vi "4Pi Drift Monitor.vi"() -> ()   [LabVIEW 2016]
uses:
  <vilib>/vision/Image Controls.llb/IMAQ Image.ctl
  4Pi Drift Monitor Controls/4Pi Drift Monitor - Notifier Type.ctl
  4Pi Drift Monitor Controls/4Pi Drift Monitor - Actions.ctl
  Hardware Configuration/Hardware Configuration Controls/Device Type.ctl
  Hardware Configuration/Hardware Configuration Controls/Device Function.ctl
panel:
  in  "CCD Offset":dbl=100.0
  in  "Offset Position Scale":dbl=2.0
  out "ROI Stack":u16[][][](array[numeric])
  out "Y (nm)":cluster{dbl, dbl, dbl, dbl}(graph)
  in  "Quit":bool
  out "Init X pos (px)":dbl[](array[numeric])
  out "Init Y pos (px)":dbl[](array[numeric])
  out "Y pos (px)":dbl[](array[numeric])
  out "X pos (px)":dbl[](array[numeric])
  in  "Frame Accumulation":i32
  in  "ROI Size":i32=7
  in  "Camera Px. Size (nm)":dbl=0.1
  in  "qd4":bool=TRUE
  in  "qd3":bool=TRUE
  in  "qd2":bool=TRUE
  in  "qd1":bool=TRUE
  out "X (nm)":cluster{dbl, dbl, dbl, dbl}(graph)
  in  "Start Monitor":bool
  # "Quadrant"
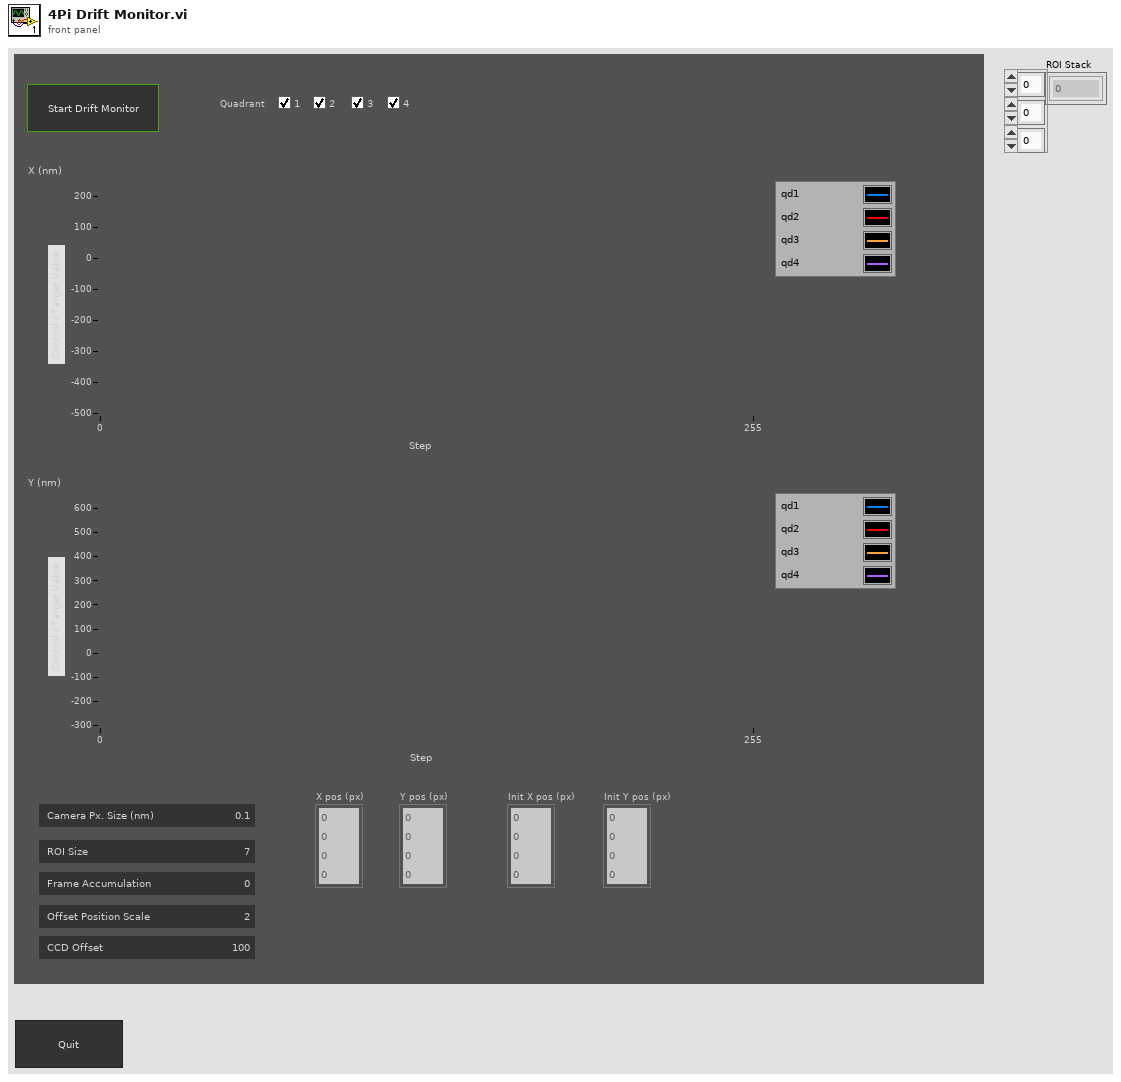
[diagram p1: front panel]
types:
  T1 = typedef "4Pi Drift Monitor - Actions.ctl" = enum16{"Idle", "Start Monitor", "Get Initial XY Pos", "Get Initial Image", "Get Image", "Get XY Position", "Update Plots", "Exit Loop", "Abort", "Quit"}
  T2 = typedef "4Pi Drift Monitor - Notifier Type.ctl" = cluster{"Action":T1, "Frame Accums.":u16, "Camera Px. Size (nm)":dbl, "QD On/Off":bool[], "Image Ref":T3[], "ROI Size":i32, "Frame Accumulation":u16, "ROI Stack":u16[][][], "Running?":bool}
  T3 = typedef "IMAQ Image.ctl" = refnum<image>
  T4 = typedef "Device Function.ctl" = enum16{"Primary", "Secondary", "Overview", "Wide Field Drift Correction", "642 nm Excitation", "560 nm Excitation", "546 nm Excitation", "488 nm Excitation", "405 nm Excitation", "Objective Drift Correction", "4Pi Objective Lock", "Objective XY", "Objective Z", "Sample XY", "Sample Coarse Z", "Sample Z", "4Pi Lower", "4Pi Upper", "Adj Cavity", "Line Scanning", "Alert"}
  T5 = typedef "Device Type.ctl" = enum16{"AOTF", "Camera", "Deformable Mirror", "Laser", "Shutter", "Stage", "Waveform", "Email"}
  T6 = typedef "4Pi DCM-2D Gaussian - Best Fit Parameters.ctl" = cluster{"Amplitude":dbl, "X Position":dbl, "Y Position":dbl, "X Width":dbl, "Y Width":dbl, "Offset":dbl}
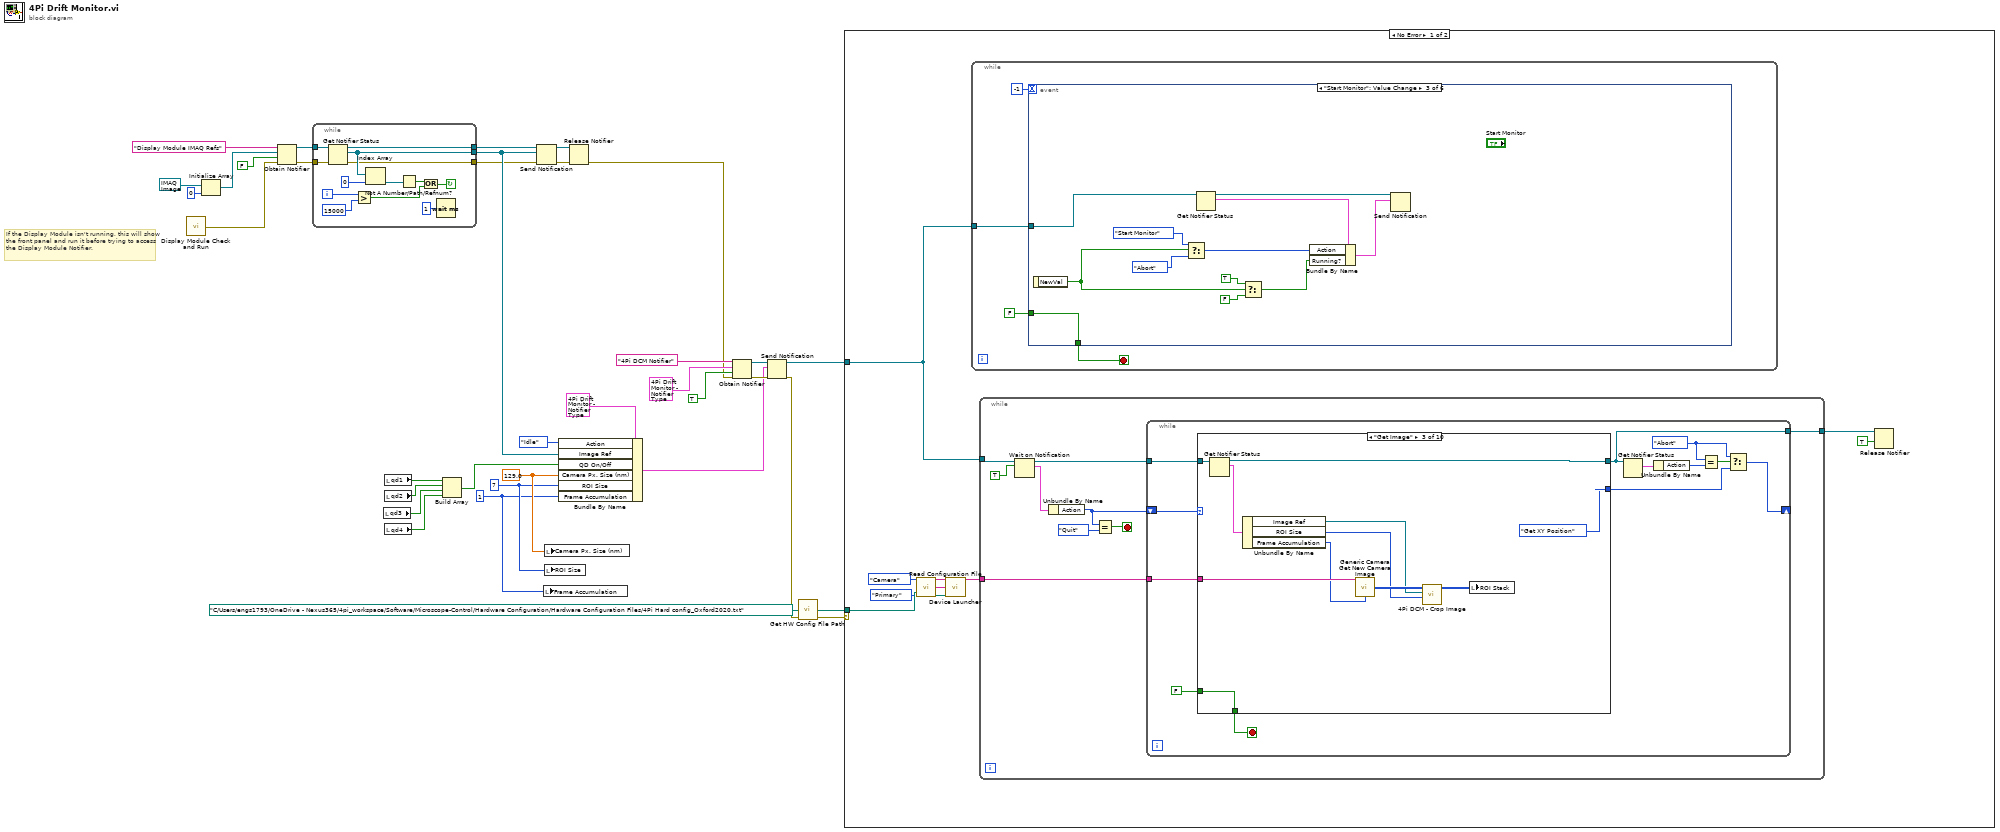
[diagram p0: block diagram]
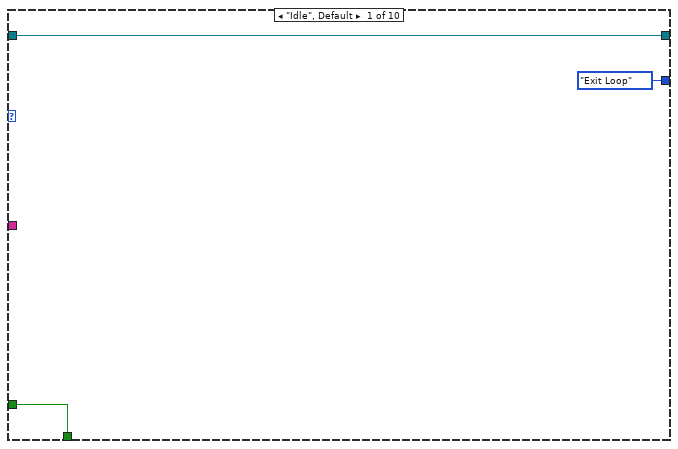
[diagram p2: hidden frame]
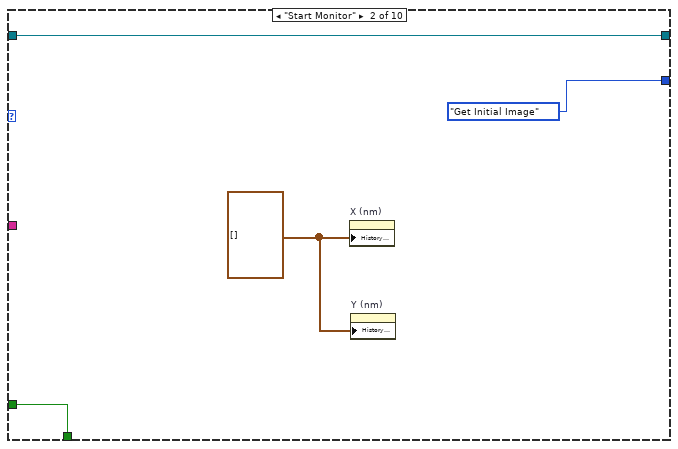
[diagram p3: hidden frame]
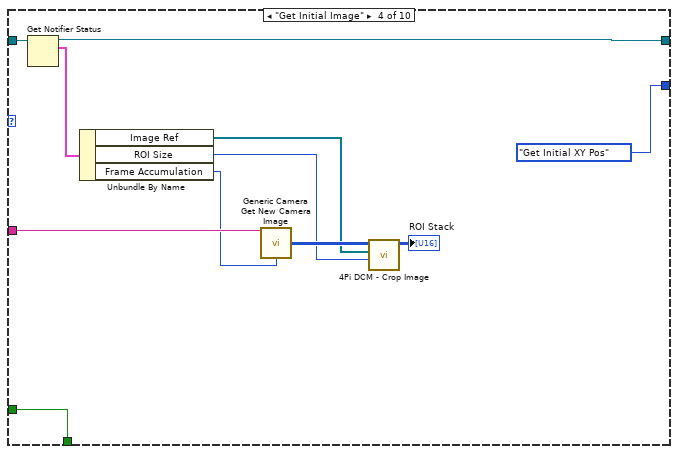
[diagram p4: hidden frame]
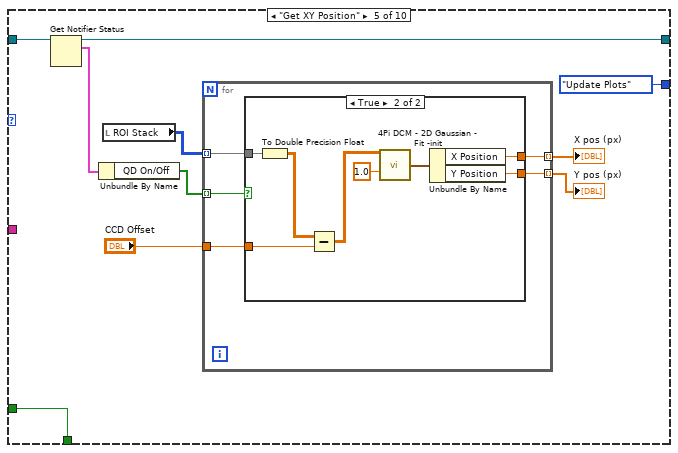
[diagram p5: hidden frame]
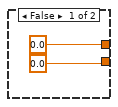
[diagram p6: hidden frame]
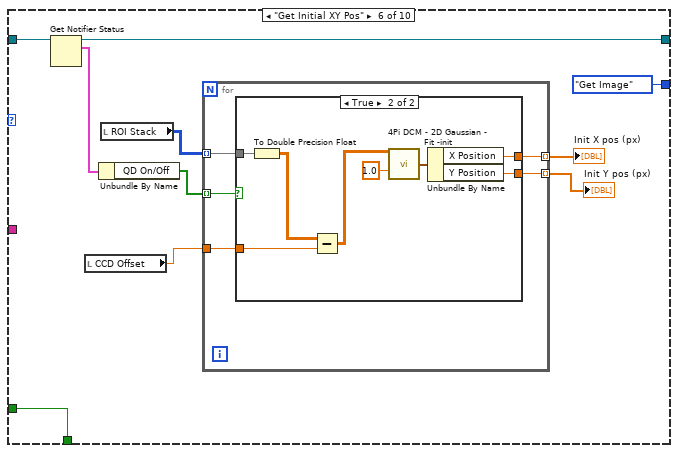
[diagram p7: hidden frame]
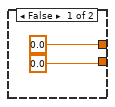
[diagram p8: hidden frame]
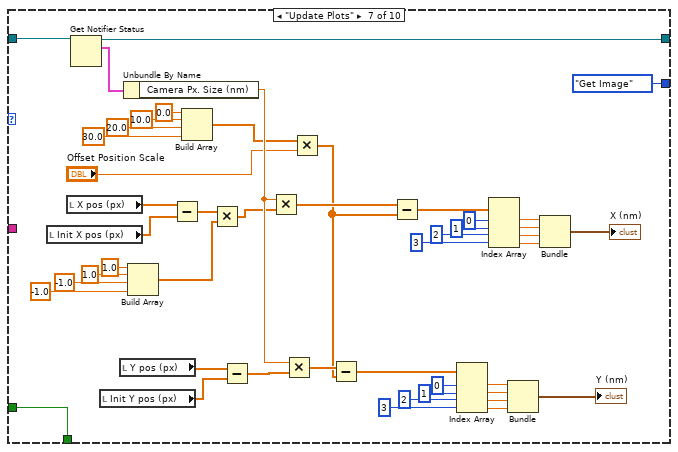
[diagram p9: hidden frame]
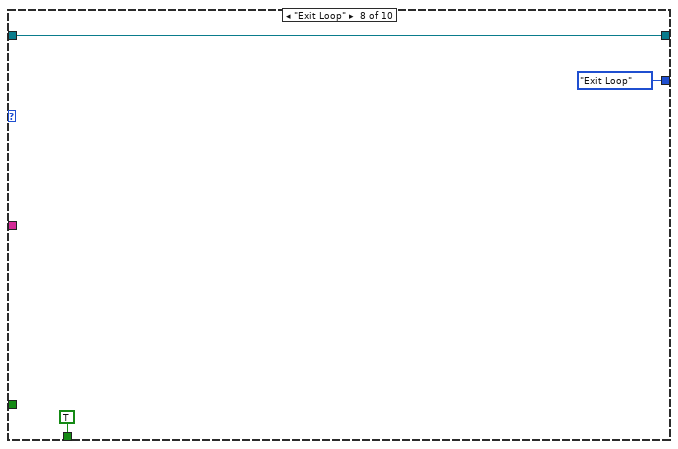
[diagram p10: hidden frame]
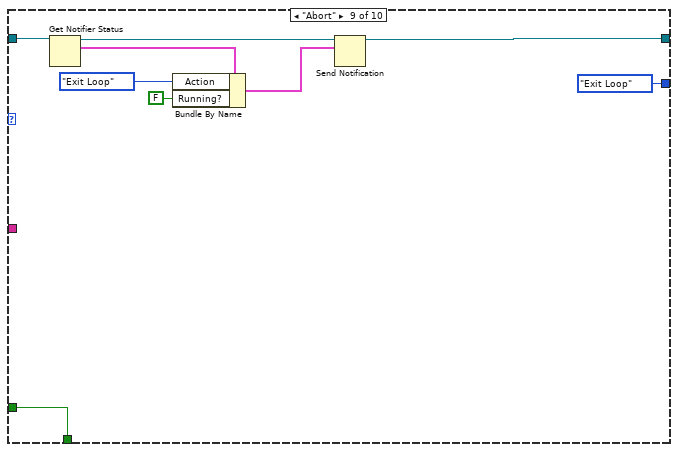
[diagram p11: hidden frame]
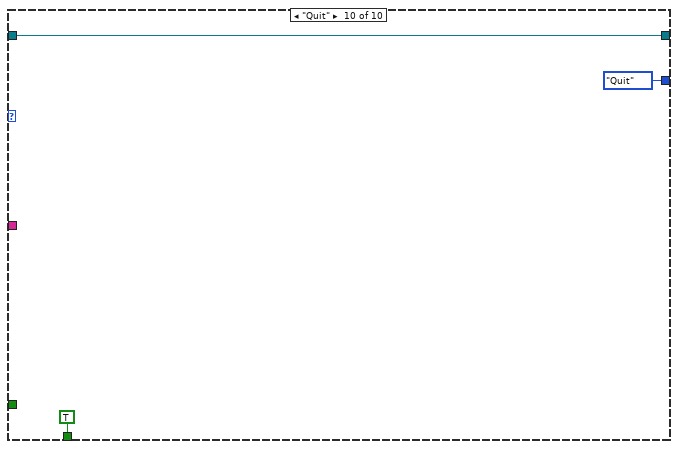
[diagram p12: hidden frame]
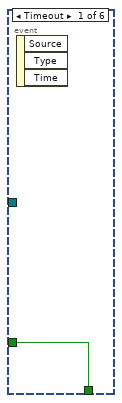
[diagram p13: hidden frame]
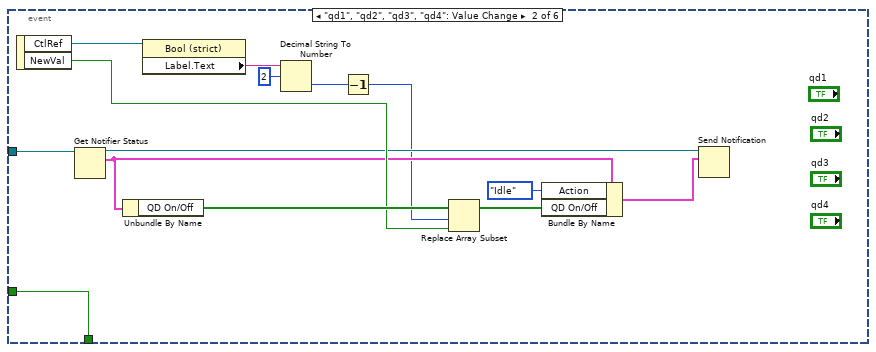
[diagram p14: hidden frame]
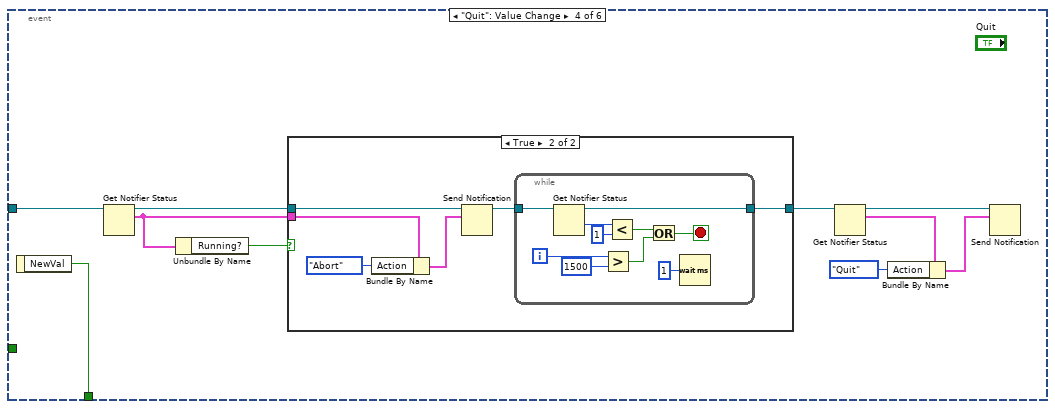
[diagram p15: hidden frame]
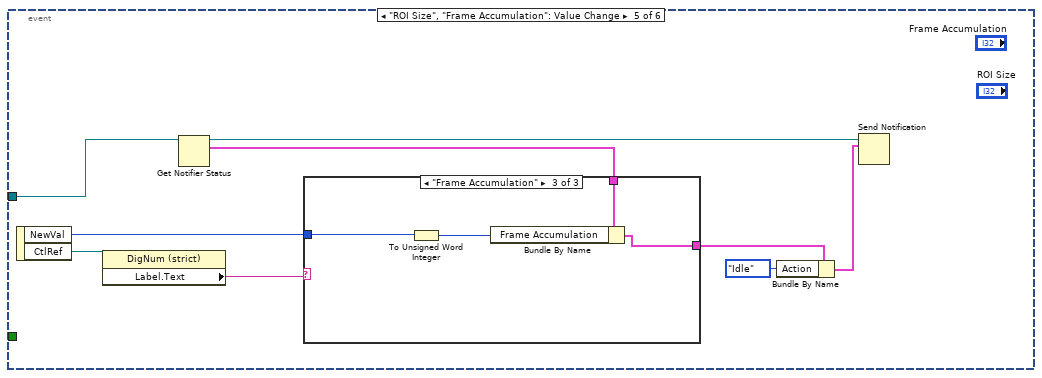
[diagram p17: hidden frame]
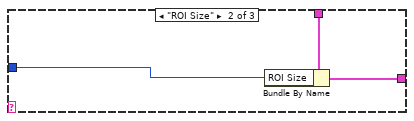
[diagram p19: hidden frame]
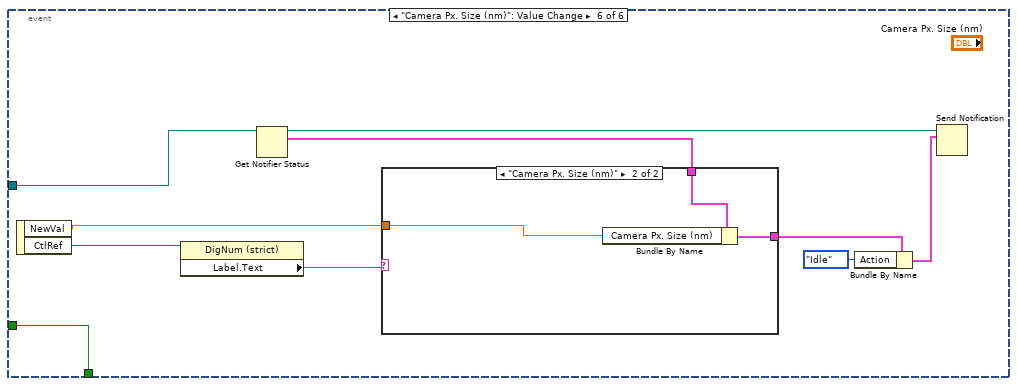
[diagram p20: hidden frame]
diagram:
  w2 = u16 1 ("Frame Accumulation")
  w3 = 7 ("ROI Size")
  w4 = 129.0 ("Camera Px. Size (nm)")
  # "If the Display Module isn't running, this will show the front panel and run it before trying to access the Display Module Notifier."
  n1 = call "Display Module Check and Run.vi"() -> ("Error"=w31:errorcluster)  [unwired: 15 in]
  n2 = Initialize Array(T3 refnum ("New Image"), 0 ("dimension size")) -> (w28:T3[])
  n3 = Obtain Notifier(name (unnamed)="Display Module IMAQ Refs", notification data type=w28, create if not found? (T)=FALSE, error in (no error)=w31) -> (notifier out=w30:refnum<notifier>, error out=w29:errorcluster)  [unwired: 1 out]
  n4 = while {
    tunnel: w30 -> [w48]
    tunnel: w29 -> [w47]
    tunnel: [w46] -> w8
    tunnel: [w45] -> w7
    tunnel: [w41] -> w6
    i -> [w40]
    stop <- w37 continue-if-true
    n5 = Get Notifier Status(notifier=w48, error in (no error)=w47) -> (notifier out=w46:refnum<notifier>, current notification=w45:T3[], error out=w41:errorcluster)  [unwired: 2 out]
    n6 = Greater?(x=w40, y=15000) -> (0:w36:bool)
    n7 = Index Array(array=w45, index=0) -> (element=w43:T3)
    n8 = Not A Number/Path/Refnum?(number/path/refnum=w43) -> (NaN/Path/Refnum?=w38:bool)
    n9 = Or(x=w38, y=w36) -> (x .or. y?=w37:bool)
    n10 = Wait (ms)(milliseconds to wait=u32 1) -> ()  [unwired: 1 out]
  }
  n11 = local read "qd3"() -> (w13:bool)
  n12 = local read "qd1"() -> (w15:bool)
  n13 = local read "qd2"() -> (w14:bool)
  n14 = local read "qd4"() -> (w12:bool)
  n15 = Build Array(w15, w14, w13, w12) -> (w11:bool[])
  n16 = Send Notification(notification=w7, notifier=w8, error in (no error)=w6) -> (notifier out=w9:refnum<notifier>, error out=w10:errorcluster)
  n17 = local write "Frame Accumulation"(w2) -> ()
  n18 = local write "Camera Px. Size (nm)"(w4) -> ()
  n19 = local write "ROI Size"(w3) -> ()
  n20 = Bundle By Name(cluster=T2 {"Action"=enum."Start Monitor", "Frame Accums."=0, "Camera Px. Size (nm)"=0.1, "QD On/Off"=[], "Image Ref"=[], "ROI Size"=0, "Frame Accumulation"=0, "ROI Stack"=[], "Running?"=FALSE} ("4Pi Drift Monitor Notifier Type"), "Action"=4Pi_Drift_Monitor_-_Actions."Idle", "Image Ref"=w7, "QD On/Off"=w11, "Camera Px. Size (nm)"=w4, "ROI Size"=w3, "Frame Accumulation"=w2) -> (w17:T2)
  n21 = Release Notifier(notifier=w9, error in (no error)=w10) -> (error out=w5:errorcluster)  [unwired: 1 in, 2 out]
  n22 = Obtain Notifier(name (unnamed)="4Pi DCM Notifier", notification data type=T2 {"Action"=enum."Start Monitor", "Frame Accums."=0, "Camera Px. Size (nm)"=0.1, "QD On/Off"=[], "Image Ref"=[], "ROI Size"=0, "Frame Accumulation"=0, "ROI Stack"=[], "Running?"=FALSE} ("4Pi Drift Monitor Notifier Type"), create if not found? (T)=TRUE, error in (no error)=w5) -> (notifier out=w25:refnum<notifier>, error out=w23:errorcluster)  [unwired: 1 out]
  n23 = Send Notification(notification=w17, notifier=w25, error in (no error)=w23) -> (notifier out=w16:refnum<notifier>, error out=w22:errorcluster)
  n24 = call "Get HW Config File Path.vi"("File Path"=path "C:/Users/engs1793/OneDrive - Nexus365/4pi_workspace/Software/Microscope-Control/Hardware Configuration/Hardware Configuration Files/4Pi Hard config_Oxford2020.txt", "Error"=w22) -> ("File Path"=w20:path, "Error"=w21:errorcluster)  [unwired: 12 in]
  n25 = case shown="No Error" w21 {
    tunnel: w20 -> [w55 _]
    tunnel: w16 -> [w51 _]
    frame No Error {
      n26 = call "Read Configuration File.vi"("Device Type"=Device_Type."Camera", "Device Function"=Device_Function."Primary", "Config File Path"=w55) -> ("Unique Notifier Name"=w56:string, "Device Ports/IDs/Channels"=w58:string[], "Device Engine Path"=w57:path)  [unwired: 9 in, 1 out]
      n27 = call "Device Launcher.vi"("Notifier Name"=w56, "Device Ports/IDs/Channels"=w58, "Device Engine Path"=w57) -> ("Notifier Name"=w52:string)  [unwired: 11 in, 1 out]
      n28 = while {
        tunnel: w51 -> [w224]
        stop <- w223 stop-if-true
        n29 = event shown="[2] \"Start Monitor\": Value Change" {
          selector: _ -> [_ _ _ _ _ _]
          dyn-events: _ -> [_ _ _ _ _ _]
          timeout: -1 -> [_ _ _ _ _ _]
          tunnel: w224 -> [_ w238 w242 w253 w285 w296]
          tunnel: [w225 w228 w245 w261 _ w305] -> w223
          tunnel: FALSE -> [w225 w228 w245 _ _ w305]
          event Timeout {
            n30 = event-data() -> ()  [unwired: 1 in, 3 out]
          }
          event "qd1", "qd2", "qd3", "qd4": Value Change {
            n31 = event-data() -> ("CtlRef"=w239:refnum<vi>, "NewVal"=w234:bool)  [unwired: 1 in]
            n32 = Get Notifier Status(notifier=w238) -> (notifier out=w230:refnum<notifier>, current notification=w233:T2)  [unwired: 1 in, 3 out]
            n33 = Unbundle By Name(w233) -> ("QD On/Off"=w237:bool[])
            n34 = property class="Bool (strict)"(reference=w239) -> ("Label.Text"=w236:string)  [unwired: 1 in, 2 out]
            n35 = Decimal String To Number(string=w236, offset=2 ("offset (0)")) -> (number=w227:i32)  [unwired: 1 in, 1 out]
            n36 = Decrement(x=w227) -> (x-1=w226:i32)
            n37 = Replace Array Subset(array=w237, new element=w234, index=w226) -> (w232:bool[])
            n38 = Bundle By Name(cluster=w233, "Action"=4Pi_Drift_Monitor_-_Actions."Idle", "QD On/Off"=w232) -> (w231:T2)
            n39 = Send Notification(notification=w231, notifier=w230) -> ()  [unwired: 1 in, 2 out]
          }
          event "Start Monitor": Value Change {
            n40 = event-data() -> ("NewVal"=w241:bool)  [unwired: 1 in]
            n41 = Select(t=4Pi_Drift_Monitor_-_Actions."Start Monitor" ("Action"), s=w241, f=4Pi_Drift_Monitor_-_Actions."Abort") -> (s? t:f=w248:T1)
            n42 = Get Notifier Status(notifier=w242) -> (notifier out=w246:refnum<notifier>, current notification=w251:T2)  [unwired: 1 in, 3 out]
            n43 = Select(t=TRUE ("Running?"), s=w241, f=FALSE) -> (s? t:f=w240:bool)
            n44 = Bundle By Name(cluster=w251, "Action"=w248, "Running?"=w240) -> (w247:T2)
            n45 = Send Notification(notification=w247, notifier=w246) -> ()  [unwired: 1 in, 2 out]
          }
          event "Quit": Value Change {
            n46 = event-data() -> ("NewVal"=w261:bool)  [unwired: 1 in]
            n47 = Get Notifier Status(notifier=w253) -> (notifier out=w256:refnum<notifier>, current notification=w254:T2)  [unwired: 1 in, 3 out]
            n48 = Unbundle By Name(w254) -> ("Running?"=w257:bool)
            n49 = case shown="True" w257 {
              tunnel: w256 -> [w262 w267]
              tunnel: [w262 w264] -> w255
              tunnel: w254 -> [_ w268]
              frame False {
              }
              frame True {
                n50 = Bundle By Name(cluster=w268, "Action"=4Pi_Drift_Monitor_-_Actions."Abort") -> (w266:T2)
                n51 = Send Notification(notification=w266, notifier=w267) -> (notifier out=w265:refnum<notifier>)  [unwired: 1 in, 1 out]
                n52 = while {
                  tunnel: w265 -> [w278]
                  tunnel: [w273] -> w264
                  i -> [w272]
                  stop <- w274 stop-if-true
                  n53 = Get Notifier Status(notifier=w278) -> (notifier out=w273:refnum<notifier>, # waiting=w277:i32)  [unwired: 1 in, 3 out]
                  n54 = Greater?(x=w272, y=1500) -> (0:w270:bool)
                  n55 = Less?(x=w277, y=1) -> (x < y?=w275:bool)
                  n56 = Or(x=w275, y=w270) -> (x .or. y?=w274:bool)
                  n57 = Wait (ms)(milliseconds to wait=u32 1) -> ()  [unwired: 1 out]
                }
              }
            }
            n58 = Get Notifier Status(notifier=w255) -> (notifier out=w259:refnum<notifier>, current notification=w260:T2)  [unwired: 1 in, 3 out]
            n59 = Bundle By Name(cluster=w260, "Action"=4Pi_Drift_Monitor_-_Actions."Quit") -> (w258:T2)
            n60 = Send Notification(notification=w258, notifier=w259) -> ()  [unwired: 1 in, 2 out]
          }
          event "ROI Size", "Frame Accumulation": Value Change {
            n61 = event-data() -> ("NewVal"=w283:i32, "CtlRef"=w287:refnum<vi>)  [unwired: 1 in]
            n62 = property class="DigNum (strict)"(reference=w287) -> ("Label.Text"=w286:string)  [unwired: 1 in, 2 out]
            n63 = Get Notifier Status(notifier=w285) -> (notifier out=w282:refnum<notifier>, current notification=w284:T2)  [unwired: 1 in, 3 out]
            n64 = case shown="\"Frame Accumulation\"" w286 {
              tunnel: w284 -> [w288 w291 w295]
              tunnel: w283 -> [_ w290 w293]
              tunnel: [w288 w289 w294] -> w281
              frame Default {
              }
              frame "ROI Size" {
                n65 = Bundle By Name(cluster=w291, "ROI Size"=w290) -> (w289:T2)
              }
              frame "Frame Accumulation" {
                n66 = To Unsigned Word Integer(number=w293) -> (unsigned 16bit integer=w292:u16)
                n67 = Bundle By Name(cluster=w295, "Frame Accumulation"=w292) -> (w294:T2)
              }
            }
            n68 = Bundle By Name(cluster=w281, "Action"=4Pi_Drift_Monitor_-_Actions."Idle") -> (w279:T2)
            n69 = Send Notification(notification=w279, notifier=w282) -> ()  [unwired: 1 in, 2 out]
          }
          event "Camera Px. Size (nm)": Value Change {
            n70 = event-data() -> ("NewVal"=w297:dbl, "CtlRef"=w298:refnum<vi>)  [unwired: 1 in]
            n71 = property class="DigNum (strict)"(reference=w298) -> ("Label.Text"=w304:string)  [unwired: 1 in, 2 out]
            n72 = Get Notifier Status(notifier=w296) -> (notifier out=w302:refnum<notifier>, current notification=w303:T2)  [unwired: 1 in, 3 out]
            n73 = case shown="\"Camera Px. Size (nm)\"" w304 {
              tunnel: w303 -> [w306 w309]
              tunnel: w297 -> [_ w308]
              tunnel: [w306 w307] -> w301
              frame Default {
              }
              frame "Camera Px. Size (nm)" {
                n74 = Bundle By Name(cluster=w309, "Camera Px. Size (nm)"=w308) -> (w307:T2)
              }
            }
            n75 = Bundle By Name(cluster=w301, "Action"=4Pi_Drift_Monitor_-_Actions."Idle") -> (w299:T2)
            n76 = Send Notification(notification=w299, notifier=w302) -> ()  [unwired: 1 in, 2 out]
          }
        }
      }
      n77 = while {
        tunnel: w52 -> [w61]
        tunnel: w51 -> [w65]
        tunnel: [w59] -> w49
        stop <- w63 stop-if-true
        n78 = Wait on Notification(notifier=w65, ignore previous (F)=TRUE) -> (notifier out=w62:refnum<notifier>, notification=w66:T2)  [unwired: 2 in, 2 out]
        n79 = Unbundle By Name(w66) -> ("Action"=w60:T1)
        n80 = Equal?(x=w60, y=4Pi_Drift_Monitor_-_Actions."Quit") -> (x = y?=w63:bool)
        n81 = while {
          tunnel: w62 -> [w79]
          tunnel: w61 -> [w78]
          shift-right: [w72] -> _
          shift-left: w60 -> [w71]
          tunnel: [w68] -> w59
          stop <- w70 stop-if-true
          w74 = 4Pi_Drift_Monitor_-_Actions."Abort" ("x")
          n82 = case shown="\"Get Image\"" w71 {
            tunnel: [w81 w86 w88 w99 w113 w138 w179 w208 w211 w218] -> w68
            tunnel: w79 -> [w81 w86 w97 w108 w118 w143 w205 w208 w217 w218]
            tunnel: w78 -> [_ _ w96 w107 _ _ _ _ _ _]
            tunnel: [4Pi_Drift_Monitor_-_Actions."Exit Loop" ("y") 4Pi_Drift_Monitor_-_Actions."Get Initial Image" ("y") 4Pi_Drift_Monitor_-_Actions."Get XY Position" ("y") 4Pi_Drift_Monitor_-_Actions."Get Initial XY Pos" ("y") 4Pi_Drift_Monitor_-_Actions."Update Plots" ("y") 4Pi_Drift_Monitor_-_Actions."Get Image" ("y") 4Pi_Drift_Monitor_-_Actions."Get Image" ("y") 4Pi_Drift_Monitor_-_Actions."Exit Loop" ("y") 4Pi_Drift_Monitor_-_Actions."Exit Loop" ("y") 4Pi_Drift_Monitor_-_Actions."Quit" ("y")] -> w73
            tunnel: [w80 w83 w89 w100 w112 w137 w178 TRUE w210 TRUE] -> w70
            tunnel: FALSE -> [w80 w83 w89 w100 w112 w137 w178 _ w210 _]
            frame "Idle", Default {
            }
            frame "Start Monitor" {
              w84 = cluster{dbl, dbl, dbl, dbl}[] [] ("History Data")
              n83 = property on="X (nm)" class="WFChart (strict)"("History Data"=w84) -> ()  [unwired: 2 in, 2 out]
              n84 = property on="Y (nm)" class="WFChart (strict)"("History Data"=w84) -> ()  [unwired: 2 in, 2 out]
            }
            frame "Get Image" {
              n85 = Get Notifier Status(notifier=w97) -> (notifier out=w88:refnum<notifier>, current notification=w91:T2)  [unwired: 1 in, 3 out]
              n86 = Unbundle By Name(w91) -> ("Image Ref"=w94:T3[], "ROI Size"=w93:i32, "Frame Accumulation"=w92:u16)
              n87 = call "Generic Camera Get New Camera Image.vi"("Camera Notifier Name"=w96, "Frames"=w92) -> ("Image - U16"=w95:u16[][])  [unwired: 11 in, 2 out]
              n88 = call "4Pi DCM - Crop Image.vi"("ROI Size"=w93, "Image Refs"=w94, "Input Image (U16)"=w95) -> ("Output Image Stack"=w87:u16[][][])  [unwired: 8 in]
              n89 = local write "ROI Stack"(w87) -> ()
            }
            frame "Get Initial Image" {
              n90 = Get Notifier Status(notifier=w108) -> (notifier out=w99:refnum<notifier>, current notification=w102:T2)  [unwired: 1 in, 3 out]
              n91 = Unbundle By Name(w102) -> ("Image Ref"=w105:T3[], "ROI Size"=w104:i32, "Frame Accumulation"=w103:u16)
              n92 = call "Generic Camera Get New Camera Image.vi"("Camera Notifier Name"=w107, "Frames"=w103) -> ("Image - U16"=w106:u16[][])  [unwired: 11 in, 2 out]
              n93 = call "4Pi DCM - Crop Image.vi"("ROI Size"=w104, "Image Refs"=w105, "Input Image (U16)"=w106) -> ("Output Image Stack"=→"ROI Stack":u16[][][])  [unwired: 8 in]
            }
            frame "Get XY Position" {
              n94 = Get Notifier Status(notifier=w118) -> (notifier out=w113:refnum<notifier>, current notification=w117:T2)  [unwired: 1 in, 3 out]
              n95 = Unbundle By Name(w117) -> ("QD On/Off"=w111:bool[])
              n96 = local read "ROI Stack"() -> (w110:u16[][][])
              n97 = for {
                tunnel: w110 -> [w123] mode=indexing
                tunnel: [w122] -> w116 mode=indexing
                tunnel: [w121] -> w115 mode=indexing
                tunnel: w111 -> [w120] mode=indexing
                tunnel: "CCD Offset" -> [w119]
                n98 = case shown="True" w120 {
                  tunnel: w123 -> [_ w133]
                  tunnel: [0.0 ("X Position") w130] -> w122
                  tunnel: [0.0 ("Y Position") w129] -> w121
                  tunnel: w119 -> [_ w127]
                  frame False {
                  }
                  frame True {
                    n99 = To Double Precision Float(number=w133) -> (double precision float=w128:dbl[][])
                    n100 = Subtract(x=w128, y=w127) -> (x-y=w126:dbl[][])
                    n101 = call "4Pi DCM - 2D Gaussian - Fit -init.vi"("Image In (DBL)"=w126, "width"=1.0) -> ("Best Fit Params"=w131:T6)  [unwired: 12 in, 1 out]
                    n102 = Unbundle By Name(w131) -> ("X Position"=w130:dbl, "Y Position"=w129:dbl)
                  }
                }
              }
              "X pos (px)" <- w116
              "Y pos (px)" <- w115
            }
            frame "Get Initial XY Pos" {
              n103 = Get Notifier Status(notifier=w143) -> (notifier out=w138:refnum<notifier>, current notification=w142:T2)  [unwired: 1 in, 3 out]
              n104 = local read "CCD Offset"() -> (w134:dbl)
              n105 = Unbundle By Name(w142) -> ("QD On/Off"=w136:bool[])
              n106 = local read "ROI Stack"() -> (w135:u16[][][])
              n107 = for {
                tunnel: w135 -> [w148] mode=indexing
                tunnel: [w147] -> w141 mode=indexing
                tunnel: [w146] -> w140 mode=indexing
                tunnel: w136 -> [w145] mode=indexing
                tunnel: w134 -> [w144]
                n108 = case shown="True" w145 {
                  tunnel: w148 -> [_ w158]
                  tunnel: [0.0 ("X Position") w155] -> w147
                  tunnel: [0.0 ("Y Position") w154] -> w146
                  tunnel: w144 -> [_ w152]
                  frame False {
                  }
                  frame True {
                    n109 = To Double Precision Float(number=w158) -> (double precision float=w153:dbl[][])
                    n110 = Subtract(x=w153, y=w152) -> (x-y=w151:dbl[][])
                    n111 = call "4Pi DCM - 2D Gaussian - Fit -init.vi"("Image In (DBL)"=w151, "width"=1.0) -> ("Best Fit Params"=w156:T6)  [unwired: 12 in, 1 out]
                    n112 = Unbundle By Name(w156) -> ("X Position"=w155:dbl, "Y Position"=w154:dbl)
                  }
                }
              }
              "Init X pos (px)" <- w141
              "Init Y pos (px)" <- w140
            }
            frame "Update Plots" {
              n113 = local read "Init X pos (px)"() -> (w202:dbl[])
              n114 = local read "X pos (px)"() -> (w203:dbl[])
              n115 = Get Notifier Status(notifier=w205) -> (notifier out=w179:refnum<notifier>, current notification=w204:T2)  [unwired: 1 in, 3 out]
              n116 = local read "Init Y pos (px)"() -> (w199:dbl[])
              n117 = local read "Y pos (px)"() -> (w200:dbl[])
              n118 = Unbundle By Name(w204) -> ("Camera Px. Size (nm)"=w198:dbl)
              n119 = Build Array(1.0 ("element"), 1.0 ("element"), -1.0 ("element"), -1.0 ("element")) -> (w160:dbl[])
              n120 = Subtract(x=w203, y=w202) -> (x-y=w161:dbl[])
              n121 = Build Array(0.0 ("element"), 10.0 ("element"), 20.0 ("element"), 30.0 ("element")) -> (w172:dbl[])
              n122 = Multiply(x=w161, y=w160) -> (x*y=w159:dbl[])
              n123 = Subtract(x=w200, y=w199) -> (x-y=w201:dbl[])
              n124 = Multiply(x=w198, y=w159) -> (x*y=w168:dbl[])
              n125 = Multiply(x=w198, y=w201) -> (x*y=w169:dbl[])
              n126 = Multiply(x=w172, y="Offset Position Scale") -> (x*y=w166:dbl[])
              n127 = Subtract(x=w169, y=w166) -> (x-y=w167:dbl[])
              n128 = Subtract(x=w168, y=w166) -> (x-y=w170:dbl[])
              n129 = Index Array(array=w167, index #1=0 ("index"), index #2=1 ("index"), index #3=2 ("index"), index #4=3 ("index")) -> (element #1=w185:dbl, element #2=w184:dbl, element #3=w183:dbl, element #4=w182:dbl)
              n130 = Index Array(array=w170, index #1=0 ("index"), index #2=1 ("index"), index #3=2 ("index"), index #4=3 ("index")) -> (element #1=w193:dbl, element #2=w192:dbl, element #3=w191:dbl, element #4=w190:dbl)
              n131 = Bundle(w185, w184, w183, w182) -> (→"Y (nm)":cluster{dbl, dbl, dbl, dbl})  [unwired: 1 in]
              n132 = Bundle(w193, w192, w191, w190) -> (→"X (nm)":cluster{dbl, dbl, dbl, dbl})  [unwired: 1 in]
            }
            frame "Exit Loop" {
            }
            frame "Abort" {
              n133 = Get Notifier Status(notifier=w217) -> (notifier out=w216:refnum<notifier>, current notification=w215:T2)  [unwired: 1 in, 3 out]
              n134 = Bundle By Name(cluster=w215, "Action"=4Pi_Drift_Monitor_-_Actions."Exit Loop", "Running?"=FALSE) -> (w214:T2)
              n135 = Send Notification(notification=w214, notifier=w216) -> (notifier out=w211:refnum<notifier>)  [unwired: 1 in, 1 out]
            }
            frame "Quit" {
            }
          }
          n136 = Get Notifier Status(notifier=w68) -> (current notification=w77:T2)  [unwired: 1 in, 4 out]
          n137 = Unbundle By Name(w77) -> ("Action"=w75:T1)
          n138 = Equal?(x=w74, y=w75) -> (x = y?=w76:bool)
          n139 = Select(t=w74, s=w76, f=w73) -> (s? t:f=w72:T1)
        }
      }
      n140 = Release Notifier(notifier=w49, force destroy? (F)=TRUE) -> ()  [unwired: 1 in, 3 out]
    }
    frame Error {
      n141 = One Button Dialog(message="Drift Monitor failed to start.") -> ()  [unwired: 1 in, 1 out]
    }
  }
